vi "MonitorTemperatureChange.vi"(6 "Monitor Temp Change? (F)":bool, 8 "error in (no error)":errorcluster, 10 "Array Out":waveform(dbl)[](array[waveform]), 11 "RoomAlert in":refnum<class "RoomAlert.lvclass">) -> (0 "error out":errorcluster, 2 "TempChangeExceedLimits":bool, 3 "RoomAlert out":refnum<class "RoomAlert.lvclass">)   [LabVIEW 2018, in "SensorPlugins.lvlib" / "RoomAlert.lvclass"]
doc: "Monitors the temperture measurements from the RoomAlert device and notifies the operator if the temperture exceeds a set threshold or the change in temperture over time is greater than a set threshold."
uses:
  RoomAlert.lvclass
  <vilib>/Utility/error.llb/Error Cluster From Error Code.vi
  <vilib>/ErrorRing/Error Ring.xnode
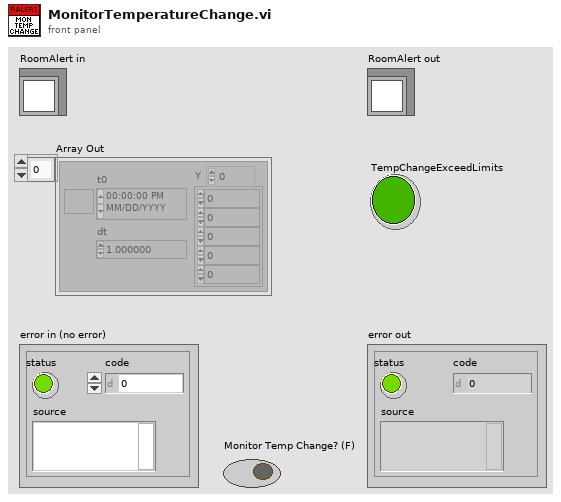
[diagram p1: front panel]
types:
  T1 = typedef "SensorPlugins.lvlib/RoomAlert.lvclass/MeasurementControls.ctl" = cluster{"Measurement RefreshTime (ms)":u32, "Measurement Name":string, "Timeout(ms)":i32, "Amber Warning Light Configuration":cluster{"Warning Temperture (Degrees C)":dbl, "Temperature Delta (Degrees C/Minute)":dbl, "Time Window (Minutes)":dbl}}
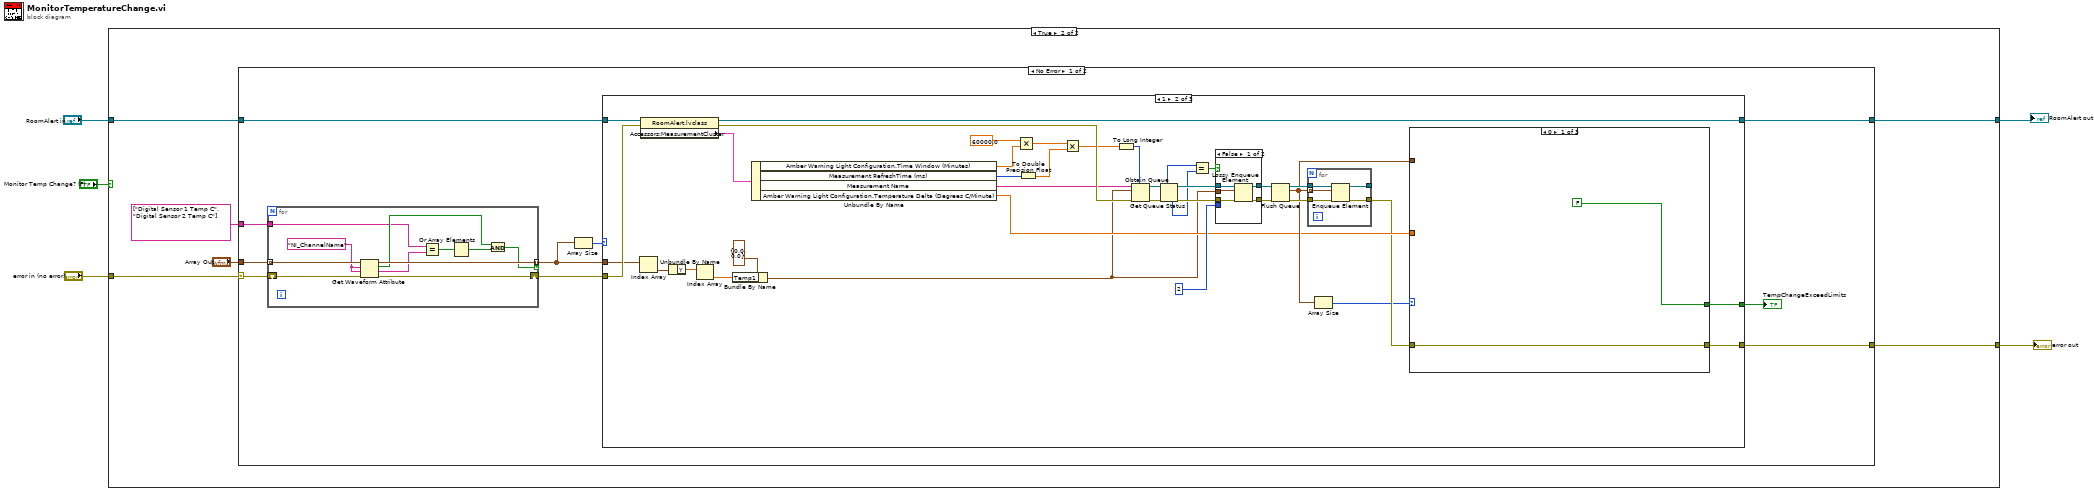
[diagram p0: block diagram]
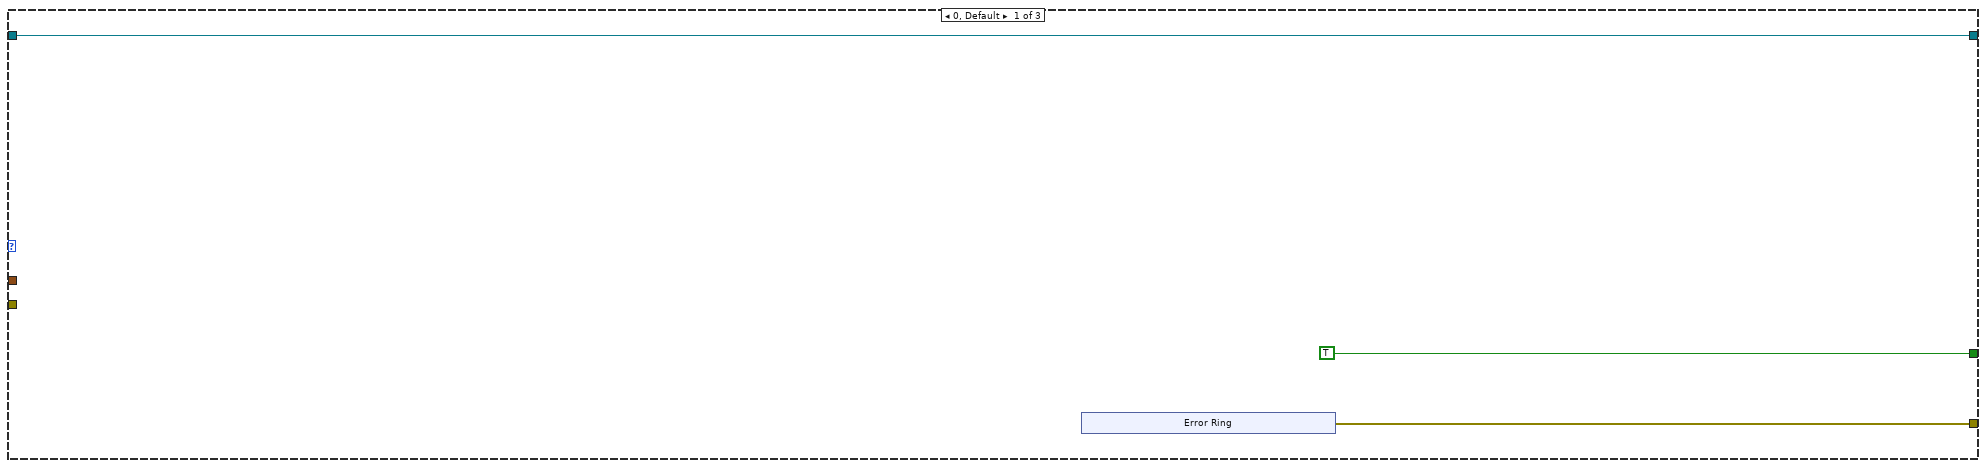
[diagram p3: hidden frame]
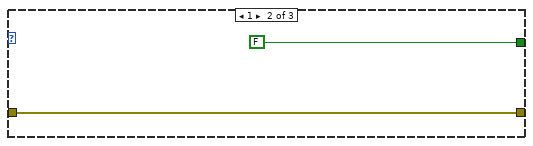
[diagram p4: hidden frame]
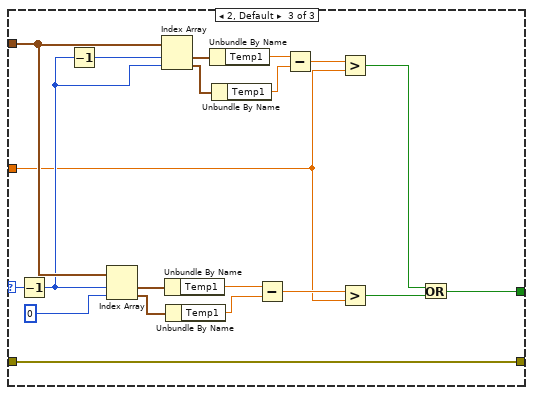
[diagram p5: hidden frame]
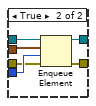
[diagram p6: hidden frame]
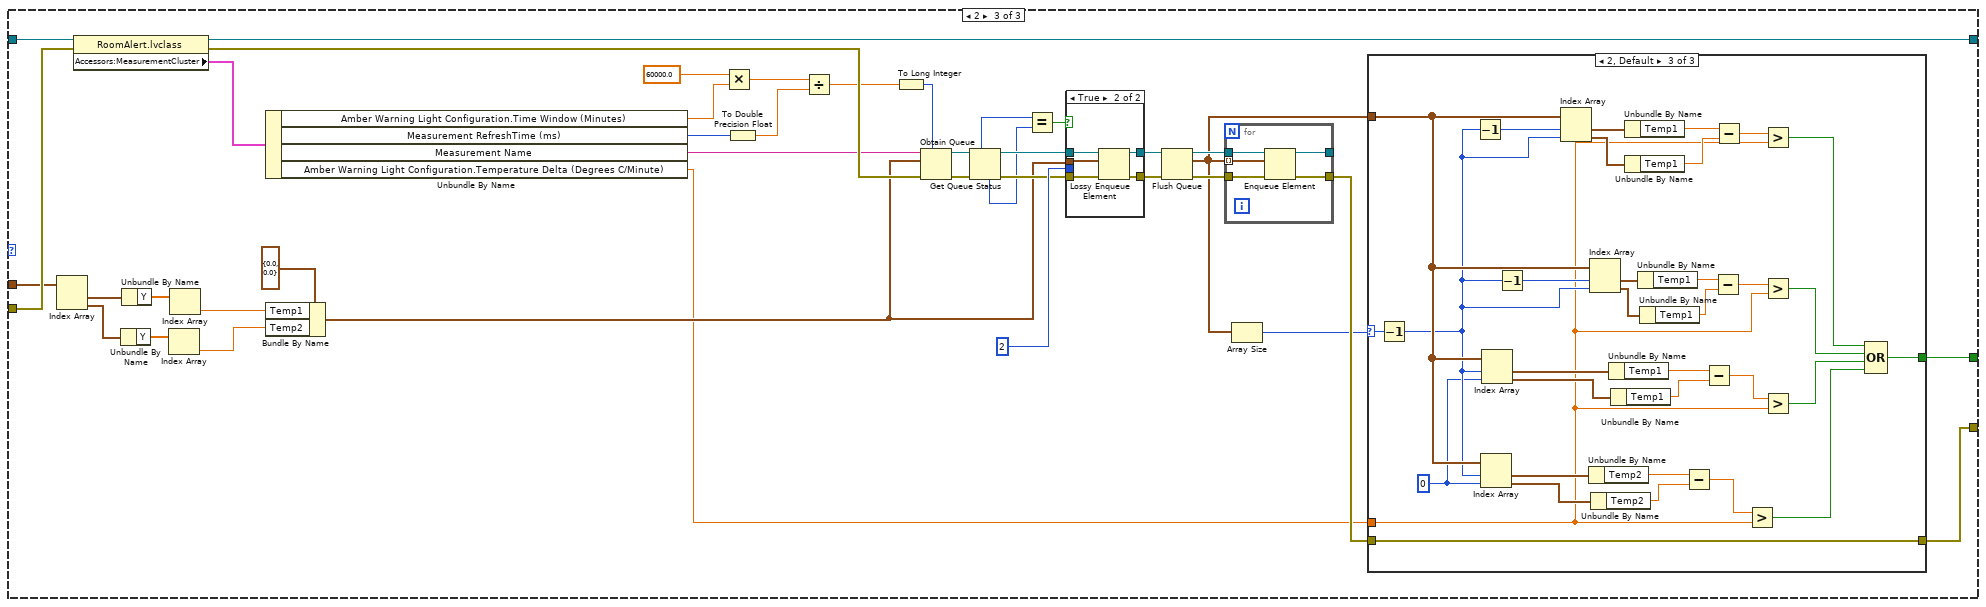
[diagram p7: hidden frame]
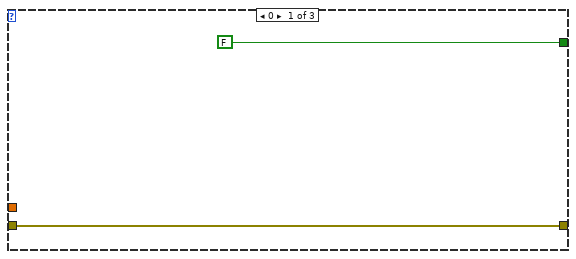
[diagram p8: hidden frame]
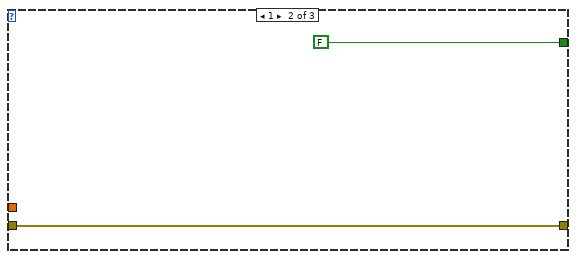
[diagram p9: hidden frame]
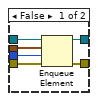
[diagram p10: hidden frame]
diagram:
  n1 = case shown="True" "Monitor Temp Change? (F)" {
    tunnel: "RoomAlert in" -> [w7 w11]
    tunnel: [w7 w10] -> w3
    tunnel: [w6 w9] -> w2
    tunnel: "error in (no error)" -> [w6 w8]
    frame False {
    }
    frame True {
      n2 = case shown="No Error" w8 {
        selector: w8 -> [w19 w214]
        tunnel: [w21 w214] -> w9
        tunnel: [w22 w213] -> w10
        tunnel: w11 -> [w23 w213]
        tunnel: "Array Out" -> [w20 _]
        tunnel: string[] ["Digital Sensor 1 Temp C", "Digital Sensor 2 Temp C"] -> [w14 _]
        frame No Error {
          n3 = for {
            tunnel: w20 -> [w34] mode=indexing
            tunnel: [w31] -> w17 mode=indexing if=w26
            shift-right: [w25] -> w18
            shift-left: w19 -> [w33]
            tunnel: w14 -> [w24]
            w32 = "NI_ChannelName" ("name")
            n4 = Get Waveform Attribute(4:w33, 5:w32, 6:w32, 7:w34) -> (0:w25:errorcluster, 1:w29:string, 2:w30:bool, 3:w31:waveform(dbl))
            n5 = Equal?(x=w24, y=w29) -> (x = y?=w28:bool[])
            n6 = Or Array Elements(Boolean array=w28) -> (logical OR=w27:bool)
            n7 = Compound Arithmetic op=AND(w30, w27) -> (w26:bool)
          }
          n8 = Array Size(array=w17) -> (size(s)=w16:i32)
          n9 = case shown="1" w16 {
            tunnel: w23 -> [w37 w79 w159]
            tunnel: [w37 w78 w158] -> w22
            tunnel: [w36 w57 w125] -> w21
            tunnel: w18 -> [_ w51 w135]
            tunnel: w17 -> [_ w49 w134]
            tunnel: [TRUE w50 w124] -> w15
            frame 0, Default {
              n10 = xnode "Error Ring"() -> ("error out"=w36:errorcluster)
            }
            frame 1 {
              n11 = Index Array(array=w49) -> (element=w47:waveform(dbl))  [unwired: 1 in]
              n12 = property class="RoomAlert.lvclass"(reference=w79, error in=w51) -> (reference out=w78:refnum<class "RoomAlert.lvclass">, error out=w77:errorcluster, "Accessors:MeasurementCluster"=w75:T1)
              n13 = Unbundle By Name(w47) -> ("Y"=w48:dbl[])
              n14 = Index Array(array=w48) -> (element=w45:dbl)  [unwired: 1 in]
              n15 = Bundle By Name(cluster=cluster{"Temp1":dbl, "Temp2":dbl} {"Temp1"=0.0, "Temp2"=0.0} ("Cluster"), "Temp1"=w45) -> (w44:cluster{"Temp1":dbl, "Temp2":dbl})
              n16 = Unbundle By Name(w75) -> ("Amber Warning Light Configuration.Time Window (Minutes)"=w60:dbl, "Measurement RefreshTime (ms)"=w53:u32, "Measurement Name"=w76:string, "Amber Warning Light Configuration.Temperature Delta (Degrees C/Minute)"=w59:dbl)
              n17 = Multiply(x=60000.0, y=w60) -> (x*y=w74:dbl)
              n18 = To Double Precision Float(number=w53) -> (double precision float=w52:dbl)
              n19 = Multiply(x=w74, y=w52) -> (x*y=w56:dbl)
              n20 = To Long Integer(number=w56) -> (32bit integer=w55:i32)
              n21 = Obtain Queue(max queue size (-1, unlimited)=w55, name (unnamed)=w76, element data type=w44, error in (no error)=w77) -> (queue out=w68:refnum<queue>, error out=w70:errorcluster)  [unwired: 1 in, 1 out]
              n22 = Get Queue Status(queue=w68, error in (no error)=w70) -> (queue out=w67:refnum<queue>, max queue size=w65:i32, error out=w69:errorcluster, # elements in queue=w66:i32)  [unwired: 1 in, 4 out]
              n23 = Equal?(x=w65, y=w66) -> (x = y?=w64:bool)
              n24 = case shown="False" w64 {
                tunnel: w44 -> [w109 w119]
                tunnel: [w113 w118] -> w73
                tunnel: [w110 w117] -> w72
                tunnel: 2 ("timeout in ms (-1)") -> [_ w116]
                tunnel: w69 -> [w112 w115]
                tunnel: w67 -> [w111 w114]
                frame False {
                  n25 = Lossy Enqueue Element(queue=w111, element=w109, error in (no error)=w112) -> (queue out=w110:refnum<queue>, error out=w113:errorcluster)  [unwired: 2 out]
                }
                frame True {
                  n26 = Enqueue Element(queue=w114, element=w119, timeout in ms (-1)=w116, error in (no error)=w115) -> (queue out=w117:refnum<queue>, error out=w118:errorcluster)  [unwired: 1 out]
                }
              }
              n27 = Flush Queue(queue=w72, error in (no error)=w73) -> (queue out=w63:refnum<queue>, remaining elements=w61:cluster{"Temp1":dbl, "Temp2":dbl}[], error out=w62:errorcluster)
              n28 = for {
                tunnel: w61 -> [w84] mode=indexing
                tunnel: w63 -> [w83]
                tunnel: w62 -> [w82]
                tunnel: [w81] -> w58
                tunnel: [w80] -> _
                n29 = Enqueue Element(queue=w83, element=w84, error in (no error)=w82) -> (queue out=w80:refnum<queue>, error out=w81:errorcluster)  [unwired: 1 in, 1 out]
              }
              n30 = Array Size(array=w61) -> (size(s)=w43:i32)
              n31 = case shown="0" w43 {
                selector: w43 -> [_ _ w97]
                tunnel: w61 -> [_ _ w105]
                tunnel: w59 -> [_ _ w90]
                tunnel: w58 -> [w86 w87 w108]
                tunnel: [w86 w87 w108] -> w57
                tunnel: [FALSE FALSE w99] -> w50
                frame 0 {
                }
                frame 1 {
                }
                frame 2, Default {
                  n32 = Decrement(x=w97) -> (x-1=w91:i32)
                  n33 = Decrement(x=w91) -> (x-1=w92:i32)
                  n34 = Index Array(array=w105, index #1=w91, index #2=0 ("index")) -> (element #1=w106:cluster{"Temp1":dbl, "Temp2":dbl}, element #2=w104:cluster{"Temp1":dbl, "Temp2":dbl})
                  n35 = Index Array(array=w105, index #1=w92, index #2=w91) -> (element #1=w107:cluster{"Temp1":dbl, "Temp2":dbl}, element #2=w96:cluster{"Temp1":dbl, "Temp2":dbl})
                  n36 = Unbundle By Name(w106) -> ("Temp1"=w102:dbl)
                  n37 = Unbundle By Name(w104) -> ("Temp1"=w101:dbl)
                  n38 = Unbundle By Name(w107) -> ("Temp1"=w94:dbl)
                  n39 = Unbundle By Name(w96) -> ("Temp1"=w93:dbl)
                  n40 = Subtract(x=w102, y=w101) -> (x-y=w98:dbl)
                  n41 = Subtract(x=w94, y=w93) -> (x-y=w95:dbl)
                  n42 = Greater?(x=w95, y=w90) -> (0:w89:bool)
                  n43 = Greater?(x=w98, y=w90) -> (0:w100:bool)
                  n44 = Or(x=w89, y=w100) -> (x .or. y?=w99:bool)
                }
              }
            }
            frame 2 {
              n45 = Index Array(array=w134) -> (element #1=w132:waveform(dbl), element #2=w130:waveform(dbl))  [unwired: 2 in]
              n46 = property class="RoomAlert.lvclass"(reference=w159, error in=w135) -> (reference out=w158:refnum<class "RoomAlert.lvclass">, error out=w157:errorcluster, "Accessors:MeasurementCluster"=w155:T1)
              n47 = Unbundle By Name(w130) -> ("Y"=w131:dbl[])
              n48 = Unbundle By Name(w132) -> ("Y"=w133:dbl[])
              n49 = Index Array(array=w131) -> (element=w127:dbl)  [unwired: 1 in]
              n50 = Index Array(array=w133) -> (element=w128:dbl)  [unwired: 1 in]
              n51 = Unbundle By Name(w155) -> ("Amber Warning Light Configuration.Time Window (Minutes)"=w141:dbl, "Measurement RefreshTime (ms)"=w137:u32, "Measurement Name"=w156:string, "Amber Warning Light Configuration.Temperature Delta (Degrees C/Minute)"=w121:dbl)
              n52 = Bundle By Name(cluster=cluster{"Temp1":dbl, "Temp2":dbl} {"Temp1"=0.0, "Temp2"=0.0} ("Cluster"), "Temp1"=w128, "Temp2"=w127) -> (w126:cluster{"Temp1":dbl, "Temp2":dbl})
              n53 = Multiply(x=60000.0, y=w141) -> (x*y=w154:dbl)
              n54 = To Double Precision Float(number=w137) -> (double precision float=w136:dbl)
              n55 = Divide(x=w154, y=w136) -> (x/y=w140:dbl)
              n56 = To Long Integer(number=w140) -> (32bit integer=w139:i32)
              n57 = Obtain Queue(max queue size (-1, unlimited)=w139, name (unnamed)=w156, element data type=w126, error in (no error)=w157) -> (queue out=w148:refnum<queue>, error out=w150:errorcluster)  [unwired: 1 in, 1 out]
              n58 = Get Queue Status(queue=w148, error in (no error)=w150) -> (queue out=w147:refnum<queue>, max queue size=w145:i32, error out=w149:errorcluster, # elements in queue=w146:i32)  [unwired: 1 in, 4 out]
              n59 = Equal?(x=w145, y=w146) -> (x = y?=w144:bool)
              n60 = case shown="True" w144 {
                tunnel: w126 -> [w207 w208]
                tunnel: [w206 w212] -> w153
                tunnel: [w205 w209] -> w152
                tunnel: 2 ("timeout in ms (-1)") -> [w204 _]
                tunnel: w149 -> [w203 w211]
                tunnel: w147 -> [w202 w210]
                frame False {
                  n61 = Enqueue Element(queue=w202, element=w207, timeout in ms (-1)=w204, error in (no error)=w203) -> (queue out=w205:refnum<queue>, error out=w206:errorcluster)  [unwired: 1 out]
                }
                frame True {
                  n62 = Lossy Enqueue Element(queue=w210, element=w208, error in (no error)=w211) -> (queue out=w209:refnum<queue>, error out=w212:errorcluster)  [unwired: 2 out]
                }
              }
              n63 = Flush Queue(queue=w152, error in (no error)=w153) -> (queue out=w143:refnum<queue>, remaining elements=w122:cluster{"Temp1":dbl, "Temp2":dbl}[], error out=w142:errorcluster)
              n64 = for {
                tunnel: w122 -> [w201] mode=indexing
                tunnel: w143 -> [w200]
                tunnel: w142 -> [w199]
                tunnel: [w198] -> w123
                tunnel: [w197] -> _
                n65 = Enqueue Element(queue=w200, element=w201, error in (no error)=w199) -> (queue out=w197:refnum<queue>, error out=w198:errorcluster)  [unwired: 1 in, 1 out]
              }
              n66 = Array Size(array=w122) -> (size(s)=w120:i32)
              n67 = case shown="2, Default" w120 {
                selector: w120 -> [_ _ w183]
                tunnel: w122 -> [_ _ w168]
                tunnel: w121 -> [_ _ w166]
                tunnel: w123 -> [w161 w163 w196]
                tunnel: [w161 w163 w196] -> w125
                tunnel: [FALSE FALSE w190] -> w124
                frame 0 {
                }
                frame 1 {
                }
                frame 2, Default {
                  w164 = 0 ("index")
                  n68 = Decrement(x=w183) -> (x-1=w167:i32)
                  n69 = Decrement(x=w167) -> (x-1=w176:i32)
                  n70 = Index Array(array=w168, index #1=w167, index #2=w164) -> (element #1=w184:cluster{"Temp1":dbl, "Temp2":dbl}, element #2=w185:cluster{"Temp1":dbl, "Temp2":dbl})
                  n71 = Index Array(array=w168, index #1=w167, index #2=w164) -> (element #1=w195:cluster{"Temp1":dbl, "Temp2":dbl}, element #2=w194:cluster{"Temp1":dbl, "Temp2":dbl})
                  n72 = Decrement(x=w167) -> (x-1=w174:i32)
                  n73 = Index Array(array=w168, index #1=w176, index #2=w167) -> (element #1=w181:cluster{"Temp1":dbl, "Temp2":dbl}, element #2=w180:cluster{"Temp1":dbl, "Temp2":dbl})
                  n74 = Unbundle By Name(w184) -> ("Temp2"=w186:dbl)
                  n75 = Index Array(array=w168, index #1=w174, index #2=w167) -> (element #1=w169:cluster{"Temp1":dbl, "Temp2":dbl}, element #2=w170:cluster{"Temp1":dbl, "Temp2":dbl})
                  n76 = Unbundle By Name(w185) -> ("Temp2"=w187:dbl)
                  n77 = Unbundle By Name(w195) -> ("Temp1"=w193:dbl)
                  n78 = Unbundle By Name(w194) -> ("Temp1"=w192:dbl)
                  n79 = Unbundle By Name(w181) -> ("Temp1"=w178:dbl)
                  n80 = Unbundle By Name(w180) -> ("Temp1"=w177:dbl)
                  n81 = Unbundle By Name(w169) -> ("Temp1"=w172:dbl)
                  n82 = Unbundle By Name(w170) -> ("Temp1"=w173:dbl)
                  n83 = Subtract(x=w186, y=w187) -> (x-y=w188:dbl)
                  n84 = Subtract(x=w193, y=w192) -> (x-y=w189:dbl)
                  n85 = Subtract(x=w172, y=w173) -> (x-y=w171:dbl)
                  n86 = Subtract(x=w178, y=w177) -> (x-y=w179:dbl)
                  n87 = Greater?(x=w188, y=w166) -> (0:w182:bool)
                  n88 = Greater?(x=w179, y=w166) -> (0:w175:bool)
                  n89 = Greater?(x=w171, y=w166) -> (0:w165:bool)
                  n90 = Greater?(x=w189, y=w166) -> (0:w191:bool)
                  n91 = Compound Arithmetic op=OR(w175, w165, w191, w182) -> (w190:bool)
                }
              }
            }
          }
          "TempChangeExceedLimits" <- w15
        }
        frame Error {
        }
      }
    }
  }
  "RoomAlert out" <- w3
  "error out" <- w2
